vi "Launcher.vi"() -> ()   [LabVIEW 2017]
doc: "JKI State Machine Objects (SMO) 1.0.0.5\nJKI - JKI\nCopyright (c) 2016, JKI"
uses:
  SystemController/Typedefs/Configuration--Cluster.ctl
  SystemController/Typedefs/CameraConfig--Cluster.ctl
  Camera/Camera_IMAQdx_class/typedefs/Configuration--Cluster.ctl
  SystemController/SystemController.lvclass
  C:/Program Files (x86)/National Instruments/LabVIEW 2017/vi.lib/JKI/JKI SMO/SMO/SMO.lvclass
  <vilib>/JKI/JKI SMO/SMO/Typedefs/SMOState --Enum.ctl
  <vilib>/JKI/JKI SMO/SMO/SMO.lvclass
  <vilib>/vision/driver/NI_Vision_Acquisition_Software.lvlib
  <vilib>/wsapi/NI_WebServices.lvlib
  Camera/Camera_IMAQdx_class/Camera_IMAQdx.lvclass
panel:
  out "picture":picture
  in  "index (0 = most recent)":i32
  in  "get image":bool
  in  "Configuration":T1={"Camera"={"Simulate Camera"=FALSE, "IMAQ Camera"={"Camera Interface Name"="cam0", "Number of Buffers"=10, "Image Name"="Face", "Image Type"=4}, "Simulated Image Folder"=path "C:/VIT/simpleImageProcessingExample/py_src/data/test1.jpg"}, "Find Eyes"=FALSE, "Acquisition Rate (ms)"=250, "Image Buffer Length"=20} {"Camera"."IMAQ Camera"."Image Type" items=["Grayscale (U8)", "Grayscale (I16)", "Grayscale (SGL)", "Complex (CSG)", "RGB (U32)", "HSL (U32)", "RGB (U64)", "Grayscale (U16)"]}
  out "error out":errorcluster
  in  "Stop":bool
  # "SMO Test Launcher"
  # "For testing the API:"
  # "For instructions on how to use the JKI State Machine Objects, examples and video tutorials, visit:\nhttp://jki.net/state-machine-objects/\n\nJKI State Machine Objects™\nhttp://jki.net/state-machine-objects/\nCopyright (C) 2005-2015, JKI <info@jki.net>\nALL RIGHTS RESERVED"
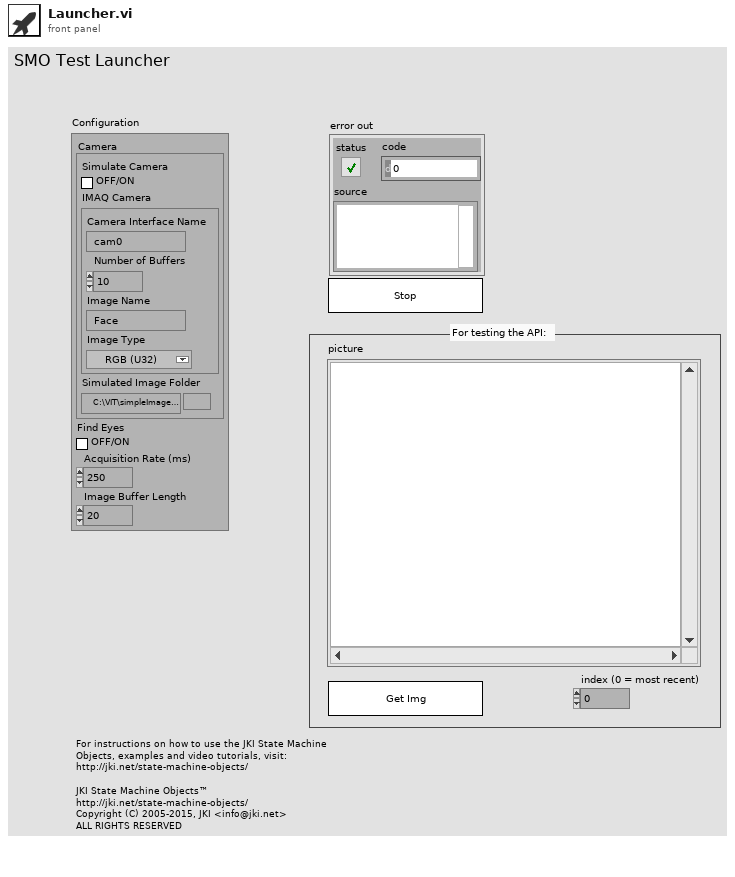
[diagram p1: front panel]
types:
  T1 = typedef "SystemController.lvclass/Configuration--Cluster.ctl" = cluster{"Camera":T2, "Find Eyes":bool, "Acquisition Rate (ms)":i32, "Image Buffer Length":i32}
  T2 = typedef "SystemController.lvclass/CameraConfig--Cluster.ctl" = cluster{"Simulate Camera":bool, "IMAQ Camera":T3, "Simulated Image Folder":path}
  T3 = typedef "Camera_IMAQdx.lvclass/Configuration--Cluster.ctl" = cluster{"Camera Interface Name":string, "Number of Buffers":u32, "Image Name":string, "Image Type":T4}
  T4 = typedef "Image Type" = u32
  T5 = cluster{"Type":u32, "Version":u32, "Flags":u32, "SerialNumberHigh":u32, "SerialNumberLow":u32, "BusType":u32, "InterfaceName":string, "VendorName":string, "ModelName":string, "CameraFileName":string, "CameraAttributeURL":string}[]
  T6 = cluster{"Type":u32, "Version":u32, "Flags":u32, "SerialNumberHigh":u32, "SerialNumberLow":u32, "BusType":u32, "InterfaceName":string, "VendorName":string, "ModelName":string, "CameraFileName":string, "CameraAttributeURL":string}
  T7 = typedef "SystemController.lvclass/PublicEvents--Cluster.ctl" = cluster{"UIClosed":refnum<user-event>}
  T8 = typedef "SMO.lvclass/Public Events.ctl" = cluster{"Error":refnum<user-event>, "State":refnum<user-event>, "Reserve State":refnum<user-event>}
  T9 = typedef "SMO.lvclass/SMOState --Enum.ctl" = enum16{"unknown", "Created", "Started", "Stopped"}
  T10 = typedef "imagedata.ctl" = cluster{"image type":i32, "image depth":i32, "image":u8[], "mask":u8[], "colors":u32[], "Rectangle":cluster{"left":i16, "top":i16, "right":i16, "bottom":i16}}
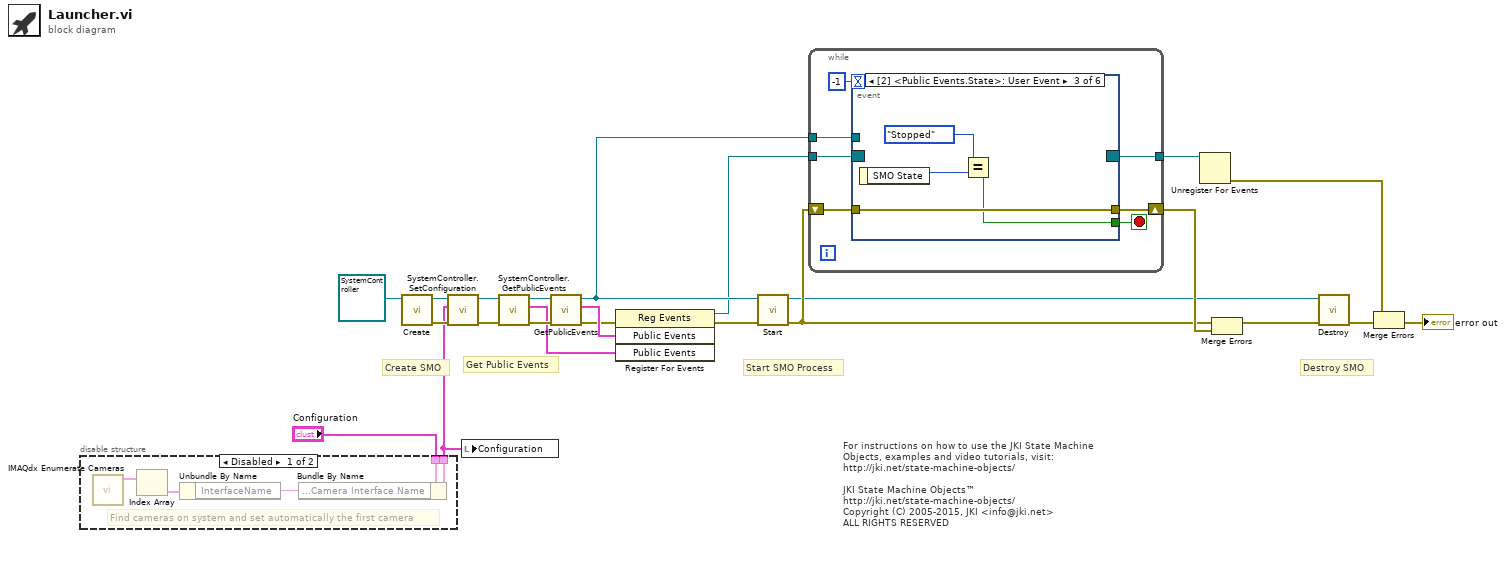
[diagram p0: block diagram]
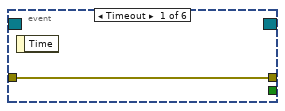
[diagram p3: hidden frame]
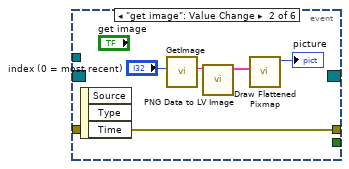
[diagram p4: hidden frame]
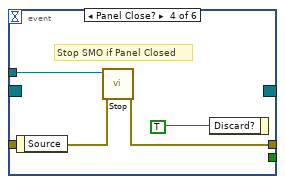
[diagram p5: hidden frame]
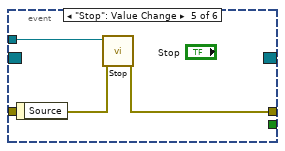
[diagram p6: hidden frame]
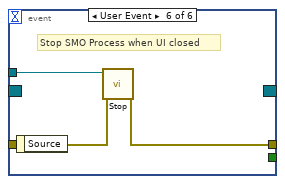
[diagram p7: hidden frame]
diagram:
  # "For instructions on how to use the JKI State Machine Objects, examples and video tutorials, visit:\nhttp://jki.net/state-machine-objects/\n\nJKI State Machine Objects™\nhttp://jki.net/state-machine-objects/\nCopyright (C) 2005-2015, JKI <info@jki.net>\nALL RIGHTS RESERVED"
  # "Get Public Events"
  # "Start SMO Process"
  # "Destroy SMO"
  # "Create SMO"
  n1 = disable-structure shown="Disabled" {
    disable-tunnel: "Configuration" -> [w26 w29]
    disable-tunnel: [w24 w29] -> w5
    frame Disabled {
      # "Find cameras on system and set automatically the first camera"
      n2 = call <vilib>:"IMAQdx Enumerate Cameras.vi"() -> ("Camera Information Array"=w28:T5)  [unwired: 10 in, 1 out]
      n3 = Index Array(array=w28) -> (element=w27:T6)  [unwired: 1 in]
      n4 = Unbundle By Name(w27) -> ("InterfaceName"=w25:string)
      n5 = Bundle By Name(cluster=w26, "Camera.IMAQ Camera.Camera Interface Name"=w25) -> (w24:T1)
    }
    frame Enabled {
    }
  }
  n6 = call <vilib>:"Create.vi"("SMO"=refnum<class "SystemController.lvclass"> refnum ("SMO.Template.lvclass")) -> ("error out"=w9:errorcluster, "SMO out"=w7:refnum<class "SystemController.lvclass">)  [unwired: 8 in, 1 out]
  n7 = call "SystemController.SetConfiguration.vi"("error in (no error)"=w9, "Configuration"=w5, "SystemController"=w7) -> ("error out"=w8:errorcluster, "SystemController out"=w3:refnum<class "SystemController.lvclass">)  [unwired: 7 in]
  n8 = local write "Configuration"(w5) -> ()
  n9 = call "SystemController.GetPublicEvents.vi"("error in (no error)"=w8, "SystemController"=w3) -> ("error out"=w4:errorcluster, "Public Events"=w1:T7, "SystemController out"=w2:refnum<class "SystemController.lvclass">)  [unwired: 7 in]
  n10 = call <vilib>:"GetPublicEvents.vi"("error in (no error)"=w4, "SMO"=w2) -> ("error out"=w11:errorcluster, "Public Events"=w12:T8, "SMO out"=w14:refnum<class "SystemController.lvclass">)  [unwired: 7 in]
  n11 = register-events(error in=w11, w12, w1) -> (reference out=w10:refnum<event-registration>, error out=w13:errorcluster)  [unwired: 1 in]
  n12 = call <vilib>:"Start.vi"("error in (no error)"=w13, "SMO"=w14) -> ("error out"=w17:errorcluster, "SMO out"=w15:refnum<class "SystemController.lvclass">)  [unwired: 8 in]
  n13 = while {
    shift-right: [w35] -> w22
    shift-left: w17 -> [w34]
    tunnel: w10 -> [w33]
    tunnel: [w32] -> w23
    tunnel: w14 -> [w31]
    stop <- w36 stop-if-true
    n14 = event shown="[2] <Public Events.State>: User Event" {
      selector: w33 -> [_ _ _ _ _ _]
      dyn-events: [_ _ _ _ _ _] -> w32
      timeout: -1 -> [_ _ _ _ _ _]
      tunnel: [_ _ w43 _ _ _] -> w36
      tunnel: w31 -> [_ _ _ w50 w53 w56]
      tunnel: [w37 w42 w46 w49 w52 w55] -> w35
      tunnel: w34 -> [w37 w42 w46 w48 w51 w54]
      event Timeout {
        n15 = event-data() -> ()  [unwired: 1 in, 1 out]
      }
      event "get image": Value Change {
        n16 = event-data() -> ()  [unwired: 1 in, 3 out]
        n17 = call "GetImage.vi"("index (0 = most recent)"="index (0 = most recent)") -> ("Img"=w40:string)  [unwired: 9 in, 1 out]
        n18 = call <vilib>:"PNG Data to LV Image.vi"("png data"=w40) -> ("image data"=w39:T10)  [unwired: 9 in, 1 out]
        n19 = call <vilib>:"Draw Flattened Pixmap.vi"("image data"=w39) -> ("new picture"=→"picture":picture)  [unwired: 8 in]
      }
      event User Event {
        n20 = event-data() -> ("SMO State"=w45:T9)  [unwired: 1 in]
        n21 = Equal?(x=SMOState_--Enum."Stopped", y=w45) -> (x = y?=w43:bool)
      }
      event Panel Close? {
        # "Stop SMO if Panel Closed"
        n22 = event-data() -> ()  [unwired: 1 in, 1 out]
        n23 = call <vilib>:"Stop.vi"("error in (no error)"=w48, "SMO"=w50) -> ("error out"=w49:errorcluster)  [unwired: 8 in, 1 out]
        n24 = event-data("Discard?"=TRUE ("OK")) -> ()  [unwired: 1 in, 1 out]
      }
      event "Stop": Value Change {
        n25 = event-data() -> ()  [unwired: 1 in, 1 out]
        n26 = call <vilib>:"Stop.vi"("error in (no error)"=w51, "SMO"=w53) -> ("error out"=w52:errorcluster)  [unwired: 8 in, 1 out]
      }
      event User Event {
        # "Stop SMO Process when UI closed"
        n27 = event-data() -> ()  [unwired: 1 in, 1 out]
        n28 = call <vilib>:"Stop.vi"("error in (no error)"=w54, "SMO"=w56) -> ("error out"=w55:errorcluster)  [unwired: 8 in, 1 out]
      }
    }
  }
  n29 = Unregister For Events(event registration refnum=w23) -> (error out=w21:errorcluster)  [unwired: 1 in]
  n30 = Merge Errors(w17, w22) -> (w16:errorcluster)
  n31 = call <vilib>:"Destroy.vi"("error in (no error)"=w16, "SMO"=w15) -> ("error out"=w19:errorcluster)  [unwired: 9 in]
  n32 = Merge Errors(w21, w19) -> (→"error out":errorcluster)
